vi "Kamarga_ME473_Project3_csvProcessing.vi"() -> ()   [LabVIEW 2018]
doc: "This VI demonstrates how a signal can be extracted from bandlimited noise using the filter VIs."
uses:
  <vilib>/Analysis/3filter.llb/Butterworth Filter (DBL).vi
  <vilib>/Utility/file.llb/Read Delimited Spreadsheet (DBL).vi
  <vilib>/Analysis/NI_AALBase.lvlib
panel:
  in  "Time Shift":dbl
  in  "P(1)":dbl
  in  "Filter Order":dbl
  out "Distance versus Time":cluster{"all rows":dbl[], dbl[]}[](graph)
  in  "Cutoff Frequency":dbl
  in  "Sampling Frequency":dbl
  in  "stop":bool
  # "ME 473 Ball on the Track Project"
  # "Filter Settings"
  # "Theoretical Plot"
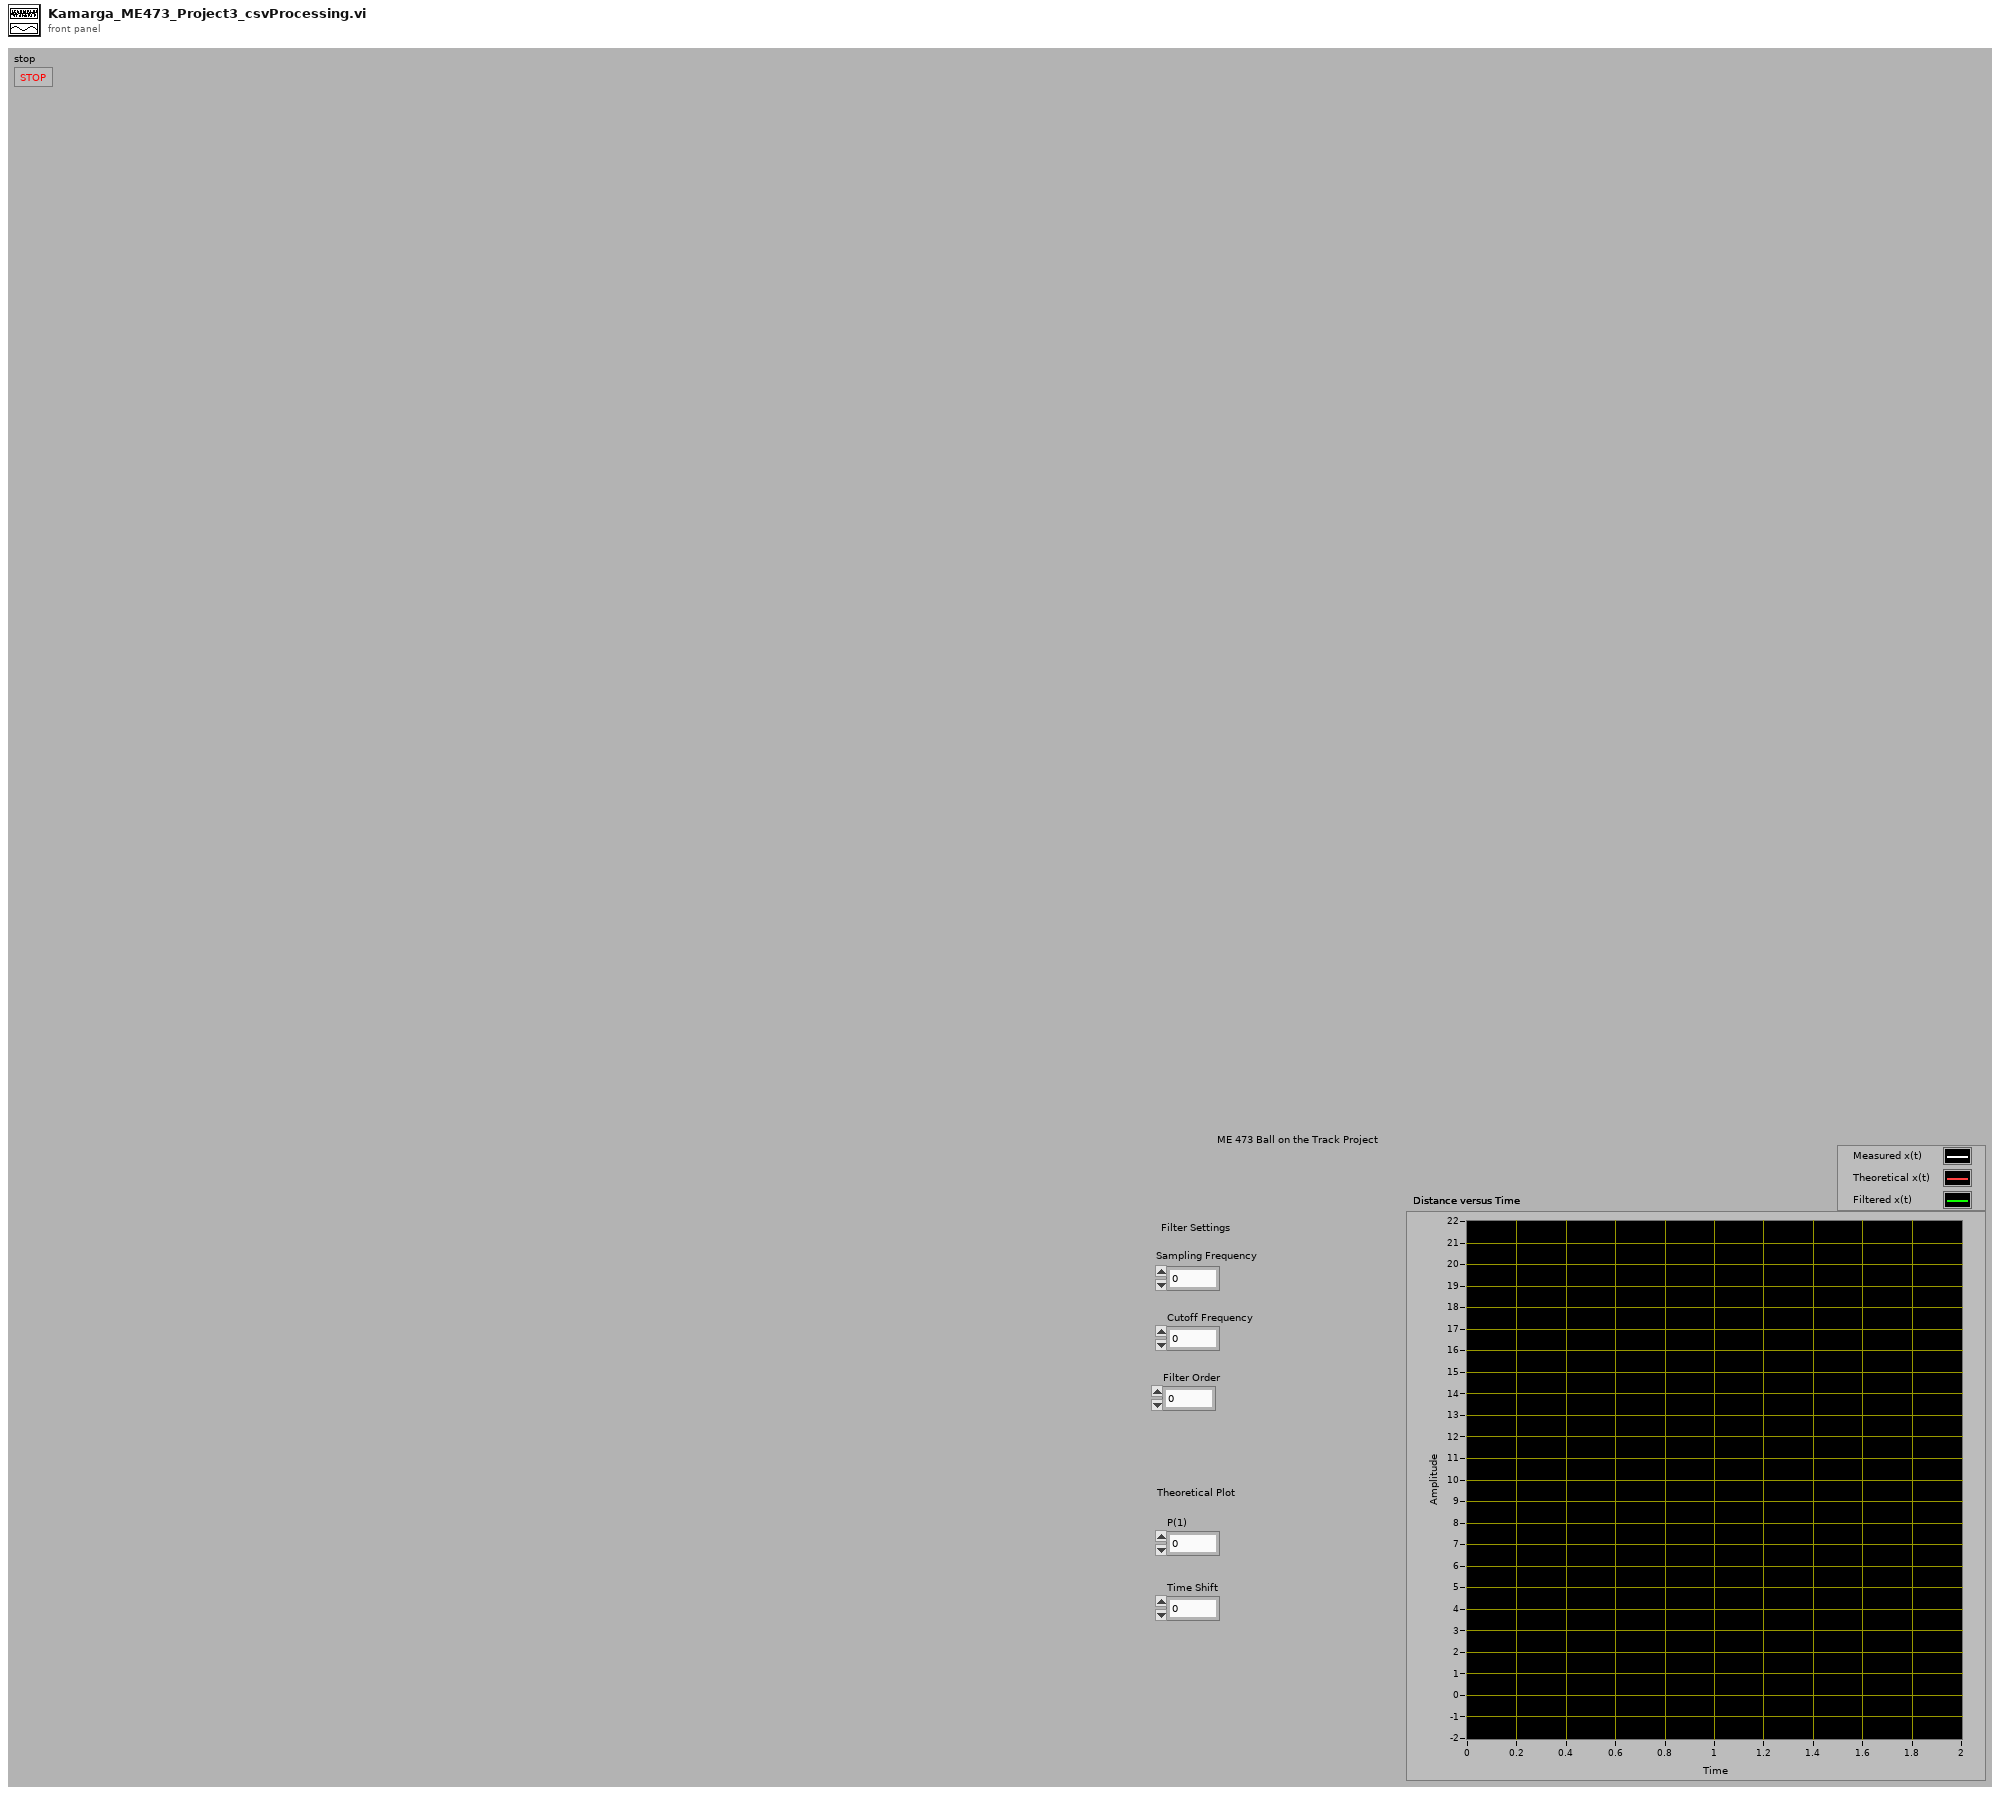
[diagram p1: front panel]
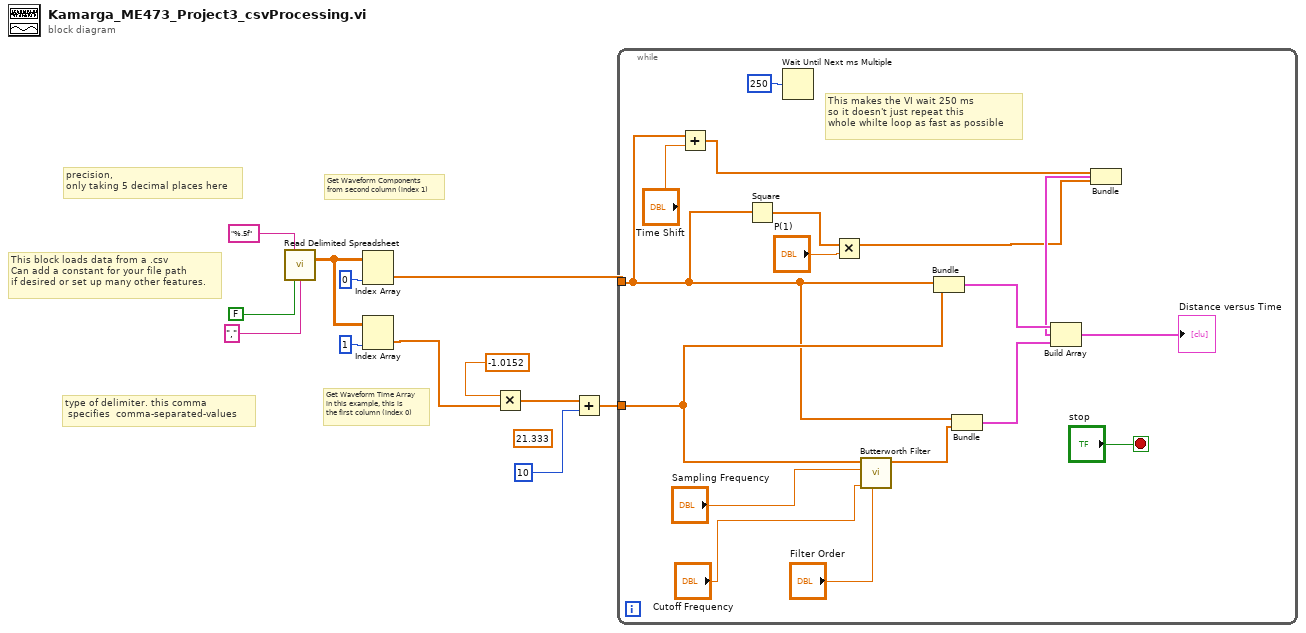
[diagram p0: block diagram]
diagram:
  (unwired) 21.333
  # "type of delimiter. this comma\n specifies  comma-separated-values"
  # "This block loads data from a .csv\nCan add a constant for your file path\nif desired or set up many other features."
  # "precision, \nonly taking 5 decimal places here"
  # "Get Waveform Components\nfrom second column (index 1)"
  # "Get Waveform Time Array\nin this example, this is\nthe first column (index 0)"
  n1 = call-poly <vilib>:"Read Delimited Spreadsheet.vi"("format (%.3f)"="%.5f", "transpose? (F)"=FALSE, "delimiter (\\t)"="," ("delimiter (\\t)")) -> ("all rows"=w12:dbl[][])  [unwired: 7 in, 5 out]
  n2 = Index Array(array=w12, index (col)=0 ("index (row)")) -> (element=w3:dbl[])  [unwired: 1 in]
  n3 = Index Array(array=w12, index (col)=1 ("index (row)")) -> (element=w6:dbl[])  [unwired: 1 in]
  n4 = Multiply(x=-1.0152, y=w6) -> (x*y=w4:dbl[])
  n5 = Add(x=w4, y=10) -> (x+y=w2:dbl[])
  n6 = while {
    tunnel: w3 -> [w15]
    tunnel: w2 -> [w23]
    stop <- "stop" stop-if-true
    # "This makes the VI wait 250 ms\nso it doesn't just repeat this \nwhole whilte loop as fast as possible"
    n7 = Add(x=w15, y="Time Shift") -> (x+y=w13:dbl[])
    n8 = Square(x=w15) -> (x^2=w19:dbl[])
    n9 = Wait Until Next ms Multiple(millisecond multiple=250) -> ()  [unwired: 1 out]
    n10 = Multiply(x=w19, y="P(1)") -> (x*y=w16:dbl[])
    n11 = call-poly <vilib>:"Butterworth Filter.vi"("order"="Filter Order", "low cutoff freq: fl"="Cutoff Frequency", "sampling freq: fs"="Sampling Frequency", "X"=w23) -> ("Filtered X"=w24:dbl[])  [unwired: 4 in, 1 out]
    n12 = Bundle("all rows"=w15, w23) -> (w22:cluster{"all rows":dbl[], dbl[]})  [unwired: 1 in]
    n13 = Bundle("all rows"=w15, "Filtered X"=w24) -> (w21:cluster{"all rows":dbl[], "Filtered X":dbl[]})  [unwired: 1 in]
    n14 = Bundle(w13, w16) -> (w17:cluster{dbl[], dbl[]})  [unwired: 1 in]
    n15 = Build Array(w22, w17, w21) -> (→"Distance versus Time":cluster{"all rows":dbl[], "Filtered X":dbl[]}[])
  }
